vi "ppanel_set_chart_properties.vi"(11 "hydraharp_panel in":refnum<class "picoharp_panel.lvclass">) -> ()   [LabVIEW 2015, in "picoharp_panel.lvclass"]
uses:
  picoharp_panel.lvclass
  UI/panel_class/panel.lvclass/panel.ctl
  UI/panel_class/panel.lvclass
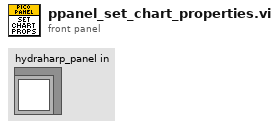
[diagram p1: front panel]
types:
  T1 = typedef "ui_plot_references.ctl" = cluster{"plots":refnum<vi>, "chart":refnum<vi>, "graph":refnum<vi>, "map":refnum<vi>, "XY Graph":refnum<vi>}
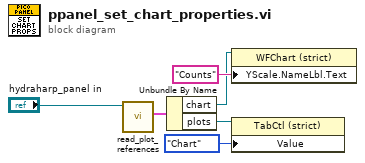
[diagram p0: block diagram]
diagram:
  n1 = call "read_plot_references.vi"("panel in"="hydraharp_panel in") -> ("plot_references"=w2:T1)  [unwired: 8 in, 2 out]
  n2 = Unbundle By Name(w2) -> ("chart"=w1:refnum<vi>, "plots"=w5:refnum<vi>)
  n3 = property class="WFChart (strict)"(reference=w1, "YScale.NameLbl.Text"="Counts" ("Y Scale.Name Label.Text")) -> ()  [unwired: 1 in, 2 out]
  n4 = property class="TabCtl (strict)"(reference=w5, "Value"=enum32{"Chart", "Graph", "Map", "XY Graph"}."Chart") -> ()  [unwired: 1 in, 2 out]
